vi "Get Oversample Factor.vi"(0 "Register Buses":refnum<class "ni579x Register Bus v1 Host.lvclass">[](array[class]), 11 "error in":errorcluster) -> (4 "Register Buses (out)":refnum<class "ni579x Register Bus v1 Host.lvclass">[](array[class]), 6 "sync.meas.oversample factor":u16[](array[numeric]), 15 "error out":errorcluster)   [LabVIEW 2012, in "ni579x Synchronization v1 Host.lvlib"]
doc: "Take a single measurement. It's possible that not all the devices will complete this sucessfully, so make sure the output Measurement Valid is true before using the measurement values."
uses:
  <instrlib>/ni579x/Synchronization/v1/Host/ni579x Synchronization v1 Host.lvlib
  <instrlib>/ni579x/Register Bus/v1/Host/ni579x Register Bus v1 Host.lvclass
  <instrlib>/ni579x/Register Bus/v1/Host/Public/Register Read Request.ctl
  <instrlib>/ni579x/Synchronization/v1/Shared/ni579x Synchronization Register Addresses.ctl
  <instrlib>/ni579x/Config/v1/Shared/Types/ni579x Register Bus Subsystem ID.ctl
  <vilib>/Utility/error.llb/Error Cluster From Error Code.vi
  <vilib>/ErrorRing/Error Ring.xnode
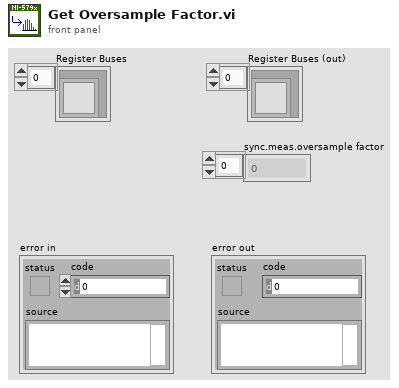
[diagram p1: front panel]
types:
  T1 = typedef "ni579x Register Bus Subsystem ID.ctl" = u8
  T2 = typedef "ni579x Synchronization Register Addresses.ctl" = enum16{"Signature", "Current Version", "Oldest Compatible Version", "Scratch Register", "sync.master", "sync.meas.enable", "sync.meas.ready", "sync.meas.arm", "sync.meas.valid", "sync.meas.value", "sync.cptr.adjust", "sync.cptr.period", "sync.meas.oversample factor"}
  T3 = typedef "ni579x Register Bus v1 Host.lvclass/Register Read Request.ctl" = cluster{"subsystem":u8, "address":u16}
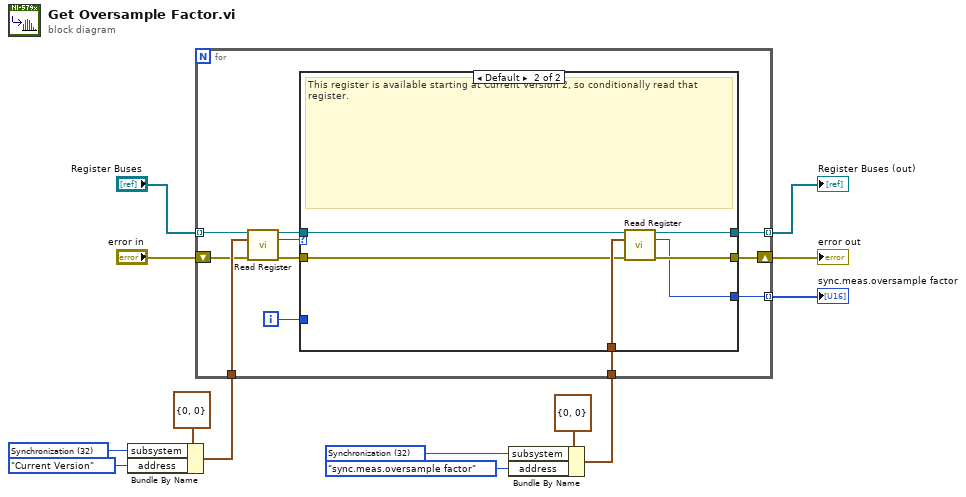
[diagram p0: block diagram]
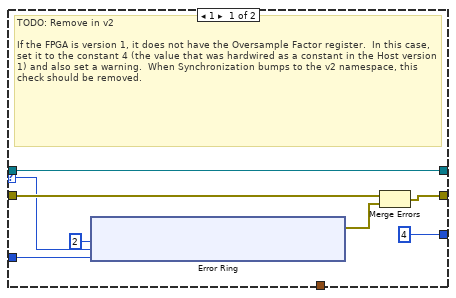
[diagram p2: hidden frame]
diagram:
  w3 = T1 32 items=["FAM Register Operation"=0, "User Command"=16, "Synchronization"=32] ("Subsystem ID")
  w10 = T1 32 items=["FAM Register Operation"=0, "User Command"=16, "Synchronization"=32] ("Subsystem ID")
  n1 = Bundle By Name(cluster=T3 {"subsystem"=0, "address"=0} ("register read request"), "subsystem"=w3, "address"=ni579x_Synchronization_Register_Addresses."Current Version" ("Synchronization Registers")) -> (w1:T3)
  n2 = Bundle By Name(cluster=T3 {"subsystem"=0, "address"=0} ("register read request"), "subsystem"=w10, "address"=ni579x_Synchronization_Register_Addresses."sync.meas.oversample factor" ("Synchronization Registers")) -> (w8:T3)
  n3 = for {
    tunnel: "Register Buses" -> [w19] mode=indexing
    tunnel: [w23] -> w6 mode=indexing
    shift-right: [w24] -> w7
    shift-left: "error in" -> [w18]
    tunnel: w8 -> [w22]
    tunnel: [w21] -> w5 mode=indexing
    tunnel: w1 -> [w20]
    i -> [w14]
    n4 = call <instrlib>:"Read Register.vi"("session in"=w19, "register read request"=w20, "error in"=w18) -> ("session out"=w16:refnum<class "ni579x Register Bus v1 Host.lvclass">, "data"=w15:u32, "error out"=w17:errorcluster)  [unwired: 10 in]
    n5 = case shown="Default" w15 {
      selector: w15 -> [w29 _]
      tunnel: [w30 w47] -> w24
      tunnel: [w26 w46] -> w23
      tunnel: w22 -> [_ w45]
      tunnel: [u32 4 ("data") w44] -> w21
      tunnel: w17 -> [w31 w43]
      tunnel: w16 -> [w26 w42]
      tunnel: w14 -> [w27 _]
      frame 1 {
        # "TODO: Remove in v2\n\nIf the FPGA is version 1, it does not have the Oversample Factor register.  In this case, set it to the constant 4 (the value that was hardwired as a constant in the Host version 1) and also set a warning.  When Synchronization bumps to the v2 namespace, this check should be removed."
        n6 = xnode ("Error Ring")("parameter 0"=2, "parameter 1"=w29, "parameter 2"=w27) -> ("error out"=w32:errorcluster)
        n7 = Merge Errors(w31, w32) -> (w30:errorcluster)
      }
      frame Default {
        # "This register is available starting at Current Version 2, so conditionally read that register."
        n8 = call <instrlib>:"Read Register.vi"("session in"=w42, "register read request"=w45, "error in"=w43) -> ("session out"=w46:refnum<class "ni579x Register Bus v1 Host.lvclass">, "data"=w44:u32, "error out"=w47:errorcluster)  [unwired: 10 in]
      }
    }
  }
  "error out" <- w7
  "Register Buses (out)" <- w6
  "sync.meas.oversample factor" <- w5
